vi "Begin.vi"(11 "Image Size":T1=enum."160x120") -> (0 "error out":errorcluster)   [LabVIEW 2011]
doc: "Called before other user functions, this VI is expected to open initial I/O refnums, load in file data, and do all program initialization. Notice that the <B>error out</B> terminal is simply used for data flow. Wiring it to other structures or subVIs ensures that this VI runs first."
uses:
  <vilib>/Rock Robotics/WPI/Camera/WPI_CameraImageSize.ctl
  <vilib>/Rock Robotics/WPI/Joystick/WPI_JoystickDeviceEnum.ctl
  <vilib>/Rock Robotics/WPI/Camera/WPI_CameraWhite Balance Values.ctl
  <vilib>/Rock Robotics/WPI/Camera/WPI_CameraExposure Values.ctl
  <vilib>/Rock Robotics/WPI/Camera/WPI_CameraFrameRate.ctl
  <vilib>/Rock Robotics/SystemInterfaces/DIO/FPGA_DIORelayChannel.ctl
  <vilib>/Rock Robotics/SystemInterfaces/DIO/FPGA_DIOChannel.ctl
  <vilib>/Rock Robotics/WPI/CAN/Jaguar/SubVIs/WPI_CANJaguar_ControlMode.ctl
  <vilib>/Rock Robotics/WPI/Solenoid/WPI_SolenoidChannel.ctl
  <vilib>/Rock Robotics/SystemInterfaces/Typedef/FPGA_TypedefAnalogModule.ctl
  <vilib>/Rock Robotics/SystemInterfaces/AI/FPGA_AIChannel.ctl
  <vilib>/Rock Robotics/SystemInterfaces/Typedef/FPGA_TypedefDigitalModule.ctl
  <vilib>/Rock Robotics/WPI/Encoder/WPI_EncoderType.ctl
  <vilib>/Rock Robotics/SystemInterfaces/DIO/FPGA_DIOPWMChannel.ctl
  <vilib>/Rock Robotics/SystemInterfaces/AI/FPGA_AIGyroChannel.ctl
  <vilib>/Rock Robotics/WPI/RobotDrive/WPI_RobotDriveOpen4MotorWithCANJaguar.vi
  <vilib>/Rock Robotics/WPI/MotorControl/WPI_MotorControlOpenCANJaguar.vi
  <vilib>/Rock Robotics/WPI/Counter/WPI_CounterDigitalInputToDigitalSource.vi
  <vilib>/Rock Robotics/WPI/Counter/WPI_CounterOpen Gear Tooth Sensor Mode.vi
  <vilib>/Rock Robotics/WPI/Solenoid/WPI_SolenoidOpenSingle.vi
  <vilib>/Rock Robotics/WPI/Compressor/WPI_CompressorGetSetRefNum.vi
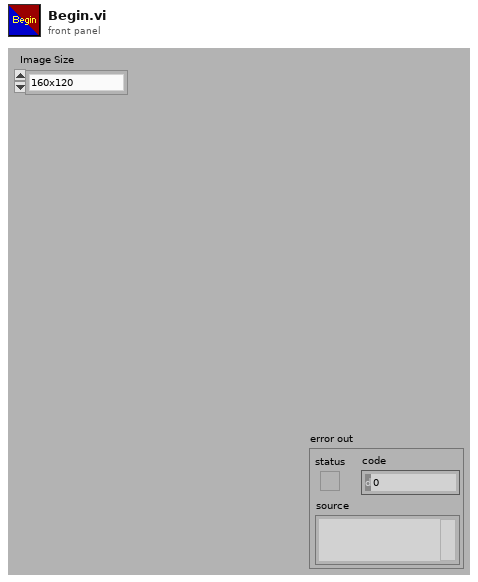
[diagram p1: front panel]
types:
  T1 = typedef "WPI_CameraImageSize.ctl" = enum16{"640x480", "320x240", "160x120"}
  T2 = typedef "WPI_SolenoidChannel.ctl" = enum8{"Solenoid 1", "Solenoid 2", "Solenoid 3", "Solenoid 4", "Solenoid 5", "Solenoid 6", "Solenoid 7", "Solenoid 8", "Invalid"}
  T3 = typedef "WPI_JoystickDeviceEnum.ctl" = enum16{"USB 1", "USB 2", "USB 3", "USB 4", "Kinect 1", "Kinect 2"}
  T4 = typedef "FPGA_AIGyroChannel.ctl" = enum8{"AI 1", "AI 2", "Invalid"}
  T5 = typedef "FPGA_DIOChannel.ctl" = enum8{"DIO 1", "DIO 2", "DIO 3", "DIO 4", "DIO 5", "DIO 6", "DIO 7", "DIO 8", "DIO 9", "DIO 10", "DIO 11", "DIO 12", "DIO 13", "DIO 14", "Invalid"}
  T6 = typedef "FPGA_DIOPWMChannel.ctl" = enum8{"PWM 1", "PWM 2", "PWM 3", "PWM 4", "PWM 5", "PWM 6", "PWM 7", "PWM 8", "PWM 9", "PWM 10", "Invalid"}
  T7 = typedef "WPI_EncoderType.ctl" = enum16{"1x", "2x", "4x"}
  T8 = typedef "FPGA_TypedefDigitalModule.ctl" = enum16{"Digital Module 1", "Digital Module 2"}
  T9 = typedef "FPGA_AIChannel.ctl" = enum8{"AI 1", "AI 2", "AI 3", "AI 4", "AI 5", "AI 6", "AI 7", "AI 8", "Invalid"}
  T10 = typedef "FPGA_TypedefAnalogModule.ctl" = enum16{"Analog Module 1", "Analog Module 2"}
  T11 = typedef "WPI_CANJaguar_ControlMode.ctl" = enum8{"Percent VBus", "Current", "Speed", "Position", "Voltage"}
  T12 = typedef "FPGA_DIORelayChannel.ctl" = enum8{"Relay 1", "Relay 2", "Relay 3", "Relay 4", "Relay 5", "Relay 6", "Relay 7", "Relay 8", "Invalid"}
  T13 = typedef "WPI_CameraFrameRate.ctl" = u32
  T14 = typedef "WPI_CameraExposure Values.ctl" = enum16{"Auto", "Flicker-free 50 Hz", "Flicker-free 60 Hz", "Hold current"}
  T15 = typedef "WPI_CameraWhite Balance Values.ctl" = enum16{"Auto", "Fixed indoor", "Fixed outdoor 1", "Fixed outdoor 2", "Fixed fluorescent 1", "Fixed fluorescent 2", "Hold current"}
  T16 = typedef "WPI_MotorControlDeviceRef.ctl" = cluster{"DeviceStatus":errorcluster, "Type":enum16{"PWM", "CAN"}, "PWM":cluster{"Digital Module":T8, "PWM Channel":T6, "DeadBand":T17}, "CAN":cluster{"Device Number":u8, "Control Mode":T11, "Semaphore":T18, "Max Vout":dbl}, "Invert":bool, "TransformRef":T19, "InvTransformRef":T19}
  T17 = typedef "WPI_PWMDeadband.ctl" = cluster{"Name":string, "maxPositivePwm":i32, "minPositivePwm":i32, "centerPwm":i32, "maxNegativePwm":i32, "minNegativePwm":i32, "angularRange":u16}
  T18 = typedef "Semaphore RefNum" = refnum<k1>
  T19 = typedef "WPI_PWMTransform_ConPane.ctl" = refnum<vi>
  T20 = typedef "WPI_DigitalInputDevRef.ctl" = cluster{"DevStatus":errorcluster, "DIO Channel":T5, "Digital Module":T8}
  T21 = typedef "WPI_JoystickDevRef.ctl" = cluster{"Device":T3}
  T22 = typedef "WPI_AnalogChannelDevRef.ctl" = cluster{"DevStatus":errorcluster, "Analog Module":T10, "Analog Channel":T9}
  T23 = typedef "WPI_RobotDriveDevRef.ctl" = cluster{"DevStatus":errorcluster, "Motors[]":T16[], "Square Inputs":bool, "Max Output":dbl, "Isochronous":bool}
  T24 = typedef "WPI_CameraDevRef.ctl" = cluster{"Camera Address":string, "CameraStatus":errorcluster, "Acquire Image Notifier":refnum<notifier>}
  T25 = typedef "WPI_SolenoidDevRef.ctl" = cluster{"DevStatus":errorcluster, "Solenoid Module":T26, "Forward Solenoid Channel":T2, "Reverse Solenoid Channel":T2}
  T26 = typedef "FPGA_TypedefSolenoidModule.ctl" = enum16{"Solenoid Module 1", "Solenoid Module 2"}
  T27 = typedef "FPGA_CounterEncoderSourceConvertionLVSourceType.ctl" = cluster{"DevStatus":errorcluster, "AnalogTriggerMode?":bool, "DigitalMode":cluster{"Digital Module":T8, "DIO Channel":T28}, "AnalogTriggerMode":cluster{"AnalogTriggerIndex":T29, "OutputType":T30}}
  T28 = typedef "FPGA_DIODigitalSourceChannel.ctl" = enum8{"DIO 1", "DIO 2", "DIO 3", "DIO 4", "DIO 5", "DIO 6", "DIO 7", "DIO 8", "DIO 9", "DIO 10", "DIO 11", "DIO 12", "DIO 13", "DIO 14", "Disabled"}
  T29 = typedef "FPGA_AnalogTriggerIndex.ctl" = enum8{"Trig 0", "Trig 1", "Trig 2", "Trig 3", "Trig 4", "Trig 5", "Trig 6", "Trig 7", "Invalid"}
  T30 = typedef "FPGA_AnalogTriggerOutType.ctl" = enum16{"InWindow", "TriggerState", "Rising", "Falling"}
  T31 = typedef "WPI_CompressorDevRef.ctl" = cluster{"DevStatus":errorcluster, "DigitalInputDevRef":T20, "RelayDevRef":T32}
  T32 = typedef "WPI_RelayDevRef.ctl" = cluster{"DevStatus":errorcluster, "Relay Channel":T12, "Digital Module":T8, "Relay Direction":T33}
  T33 = typedef "WPI_RelayDirection.ctl" = enum16{"Both directions", "Forward only", "Reverse only"}
  T34 = typedef "WPI_GyroDevRef.ctl" = cluster{"DevStatus":errorcluster, "Analog Module":T10, "Analog Channel":T9, "Offset":dbl, "Gain (VoltsPerDegree/Second)":dbl}
  T35 = typedef "WPI_CounterDevRef.ctl" = cluster{"DevStatus":errorcluster, "CntIndex":T36}
  T36 = typedef "FPGA_CounterCtrSystemIndex.ctl" = enum8{"Ctr 0", "Ctr 1", "Ctr 2", "Ctr 3", "Ctr 4", "Ctr 5", "Ctr 6", "Ctr 7", "Invalid"}
  T37 = typedef "WPI_ServoDeviceRef.ctl" = cluster{"DeviceStatus":errorcluster, "Digital Module":T8, "PWM Channel":T6, "DeadBand":T17}
  T38 = typedef "WPI_EncoderDevRef.ctl" = cluster{"DevStatus":errorcluster, "EncoderIndex":T39, "CounterIndex":T36, "DistancePerCount":dbl, "Decoding Type":T7}
  T39 = typedef "FPGA_EncoderIdx.ctl" = enum8{"Enc 0", "Enc 1", "Enc 2", "Enc 3", "Invalid"}
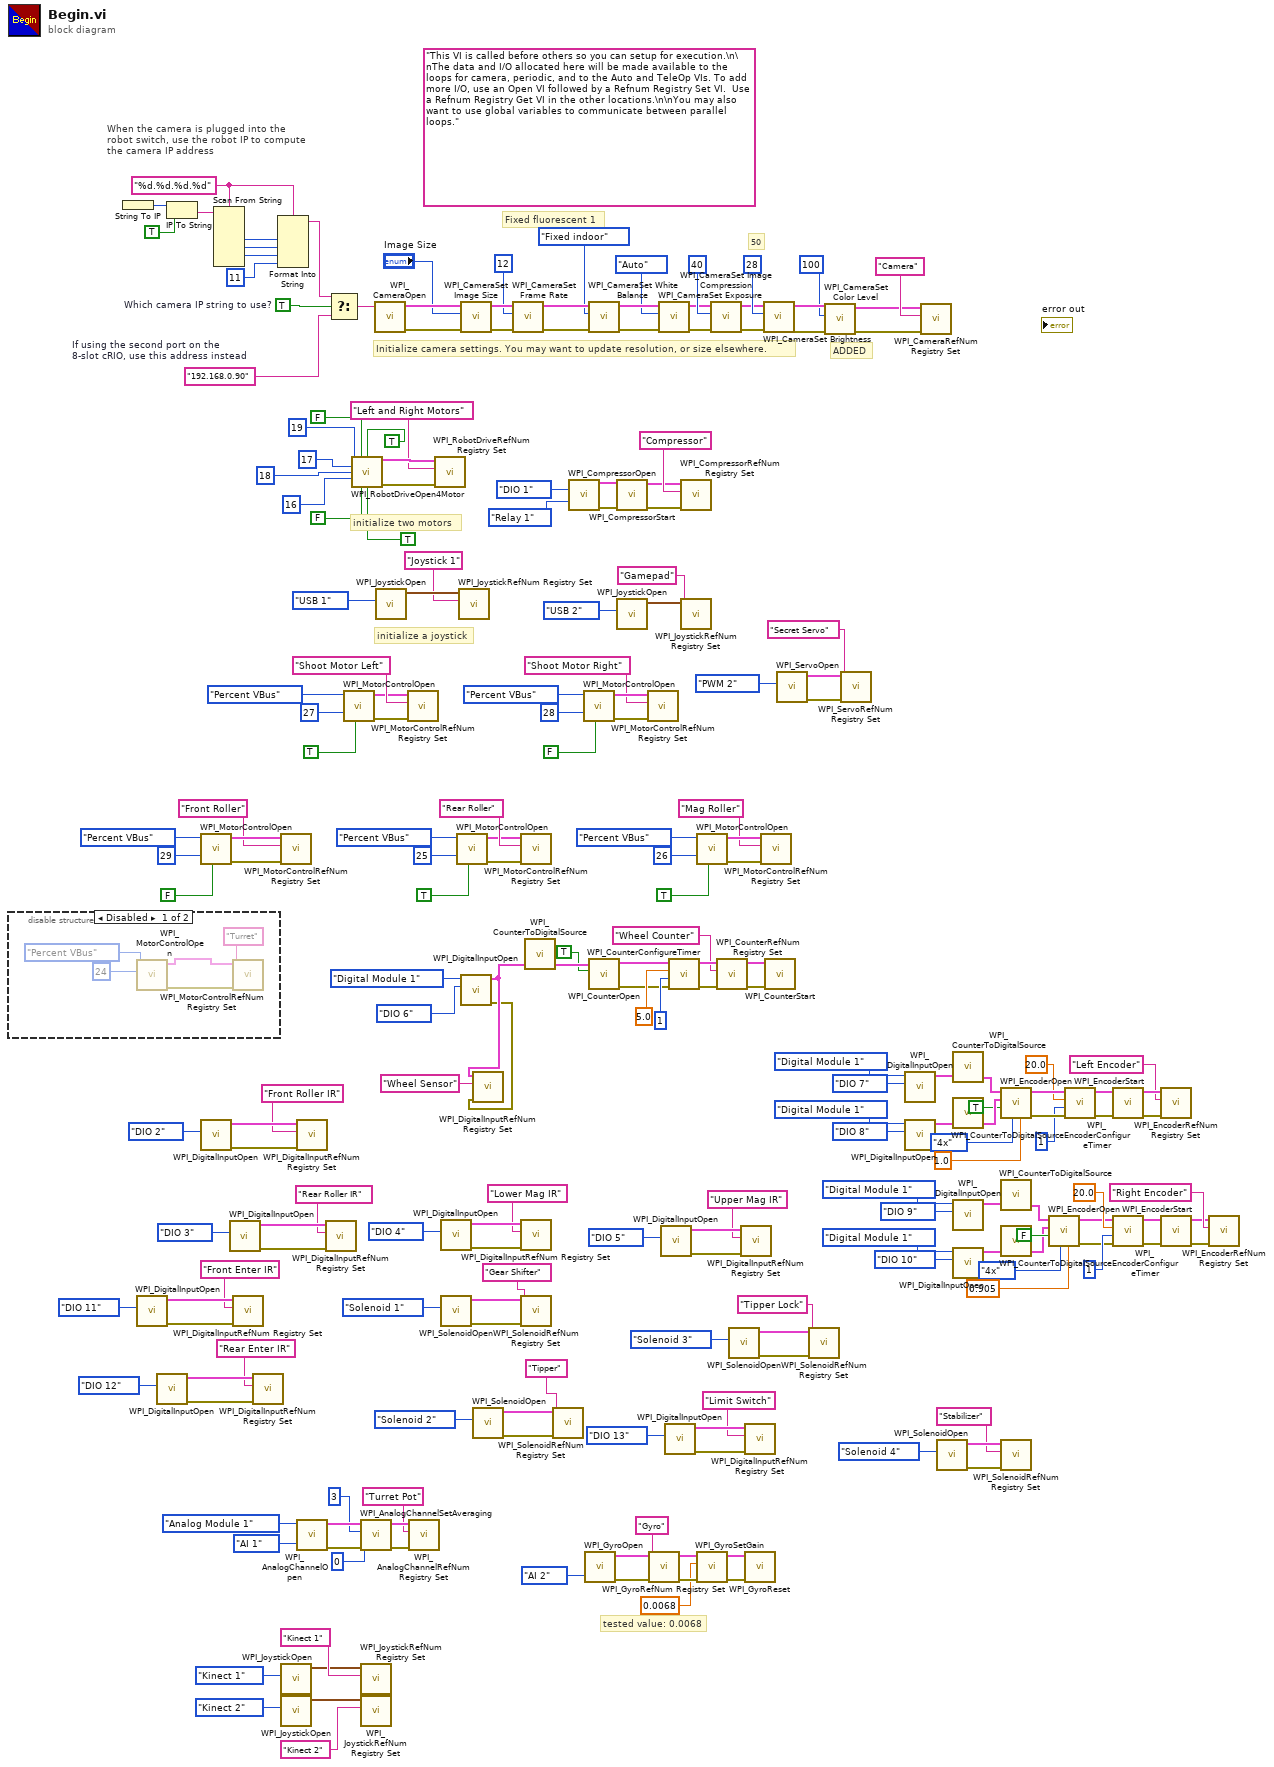
[diagram p0: block diagram]
diagram:
  w185 = TRUE  # Which camera IP string to use?
  w189 = "%d.%d.%d.%d" ("format string")
  (unwired) "This VI is called before others so you can setup for execution.\n\nThe data and I/O allocated here will be made available to the loops for camera, periodic, and to the Auto and TeleOp VIs. To add more I/O, use an Open VI followed by a Refnum Registry Set VI.  Use a Refnum Registry Get VI in the other locations.\n\nYou may also want to use global variables to communicate between parallel loops."
  w186 = "192.168.0.90"  # If using the second port on the 8-slot cRIO, use this address instead
  # "ADDED"
  # "50"
  # "Fixed fluorescent 1"
  # "tested value: 0.0068"
  # "initialize two motors"
  # "When the camera is plugged into the\nrobot switch, use the robot IP to compute\nthe camera IP address"
  # "initialize a joystick"
  # "Initialize camera settings. You may want to update resolution, or size elsewhere."
  n1 = disable-structure shown="Disabled" {
    frame Disabled {
      n2 = call-poly <vilib>:"WPI_MotorControlOpen.vi"("Device Number"=u8 24, "Control Mode"=WPI_CANJaguar_ControlMode."Percent VBus") -> ("error out"=w219:errorcluster, "MotorControlDeviceRef"=w221:T16)  [unwired: 8 in]
      n3 = call <vilib>:"WPI_MotorControlRefNum Registry Set.vi"("error in (no error)"=w219, "refnum name"="Turret", "MotorControlDevRef"=w221) -> ()  [unwired: 7 in, 2 out]
    }
    frame Enabled {
    }
  }
  n4 = String To IP() -> (0:w196:u32)  [unwired: 1 in]
  n5 = call <vilib>:"WPI_DigitalInputOpen.vi"("DIO Channel"=FPGA_DIOChannel."DIO 11") -> ("error out"=w33:errorcluster, "DigitalInputDevRef"=w36:T20)  [unwired: 9 in]
  n6 = call <vilib>:"WPI_DigitalInputOpen.vi"("DIO Channel"=FPGA_DIOChannel."DIO 12") -> ("error out"=w29:errorcluster, "DigitalInputDevRef"=w32:T20)  [unwired: 9 in]
  n7 = IP To String(1:TRUE ("dot notation? (F)"), 2:w196) -> (0:w194:string)
  n8 = call-poly <vilib>:"WPI_MotorControlOpen.vi"("Invert"=FALSE, "Device Number"=u8 29, "Control Mode"=WPI_CANJaguar_ControlMode."Percent VBus") -> ("error out"=w148:errorcluster, "MotorControlDeviceRef"=w149:T16)  [unwired: 7 in]
  n9 = call <vilib>:"WPI_DigitalInputOpen.vi"("DIO Channel"=FPGA_DIOChannel."DIO 2") -> ("error out"=w106:errorcluster, "DigitalInputDevRef"=w118:T20)  [unwired: 9 in]
  n10 = Scan From String(format string=w189, input string=w194) -> (output 1=w193:i32, output 2=w192:i32, output 3=w191:i32)  [unwired: 7 in, 3 out]
  n11 = call <vilib>:"WPI_DigitalInputOpen.vi"("DIO Channel"=FPGA_DIOChannel."DIO 3") -> ("error out"=w105:errorcluster, "DigitalInputDevRef"=w115:T20)  [unwired: 9 in]
  n12 = call <vilib>:"WPI_DigitalInputRefNum Registry Set.vi"("error in (no error)"=w33, "refnum name"="Front Enter IR", "DigitalInputDevRef"=w36) -> ()  [unwired: 7 in, 2 out]
  n13 = call <vilib>:"WPI_DigitalInputRefNum Registry Set.vi"("error in (no error)"=w29, "refnum name"="Rear Enter IR", "DigitalInputDevRef"=w32) -> ()  [unwired: 7 in, 2 out]
  n14 = Format Into String(format string=w189, w193, w192, w191, 11 ("Compression")) -> (resulting string=w187:string)  [unwired: 2 in, 1 out]
  n15 = call <vilib>:"WPI_MotorControlRefNum Registry Set.vi"("error in (no error)"=w148, "refnum name"="Front Roller", "MotorControlDevRef"=w149) -> ()  [unwired: 7 in, 2 out]
  n16 = call <vilib>:"WPI_JoystickOpen.vi"("JoystickDevice"=WPI_JoystickDeviceEnum."Kinect 1") -> ("JoystickDevRef"=w12:T21)  [unwired: 10 in]
  n17 = call <vilib>:"WPI_JoystickOpen.vi"("JoystickDevice"=WPI_JoystickDeviceEnum."Kinect 2") -> ("JoystickDevRef"=w15:T21)  [unwired: 10 in]
  n18 = call <vilib>:"WPI_DigitalInputRefNum Registry Set.vi"("error in (no error)"=w106, "refnum name"="Front Roller IR", "DigitalInputDevRef"=w118) -> ()  [unwired: 7 in, 2 out]
  n19 = call <vilib>:"WPI_AnalogChannelOpen.vi"("Analog Channel"=FPGA_AIChannel."AI 1", "Analog Module (Module 1)"=FPGA_TypedefAnalogModule."Analog Module 1") -> ("error out"=w86:errorcluster, "AIDeviceRef"=w87:T22)  [unwired: 8 in]
  n20 = call <vilib>:"WPI_DigitalInputRefNum Registry Set.vi"("error in (no error)"=w105, "refnum name"="Rear Roller IR", "DigitalInputDevRef"=w115) -> ()  [unwired: 7 in, 2 out]
  n21 = Select(t=w187, s=w185, f=w186) -> (s? t:f=w188:string)
  n22 = call-poly <vilib>:"WPI_MotorControlOpen.vi"("Invert"=TRUE, "Device Number"=u8 27, "Control Mode"=WPI_CANJaguar_ControlMode."Percent VBus") -> ("error out"=w164:errorcluster, "MotorControlDeviceRef"=w163:T16)  [unwired: 7 in]
  n23 = call-poly <vilib>:"WPI_RobotDriveOpen4Motor.vi"("Rear Left Motor"=u8 19, "Rear Left Motor Inverted"=FALSE, "Rear Right Motor Inverted"=TRUE ("Rear Left Motor Inverted"), "Rear Right Motor"=u8 17, "Front Left Motor"=u8 18, "Front Right Motor"=u8 16, "Front Left Motor Inverted"=FALSE, "Front Right Motor Inverted"=TRUE) -> ("RobotDriveDevRef"=w184:T23, "error out"=w182:errorcluster)  [unwired: 6 in]
  n24 = call <vilib>:"WPI_AnalogChannelSetAveraging.vi"("error in (no error)"=w86, "OversampleBits"=u8 0, "AverageBits"=u8 3, "AIDeviceRef"=w87) -> ("error out"=w83:errorcluster, "AIDeviceRef"=w82:T22)  [unwired: 6 in]
  n25 = call <vilib>:"WPI_JoystickRefNum Registry Set.vi"("refnum name"="Kinect 1", "JoystickDevRef"=w12) -> ()  [unwired: 8 in, 2 out]
  n26 = call <vilib>:"WPI_JoystickRefNum Registry Set.vi"("refnum name"="Kinect 2", "JoystickDevRef"=w15) -> ()  [unwired: 8 in, 2 out]
  n27 = call <vilib>:"WPI_CameraOpen.vi"("Camera Address"=w188) -> ("error out"=w207:errorcluster, "CameraDevRef"=w208:T24)  [unwired: 1 in, 8 out]
  n28 = call <vilib>:"WPI_JoystickOpen.vi"("JoystickDevice"=WPI_JoystickDeviceEnum."USB 1") -> ("JoystickDevRef"=w217:T21)  [unwired: 10 out]
  n29 = call <vilib>:"WPI_MotorControlRefNum Registry Set.vi"("error in (no error)"=w164, "refnum name"="Shoot Motor Left", "MotorControlDevRef"=w163) -> ()  [unwired: 7 in, 2 out]
  n30 = call <vilib>:"WPI_AnalogChannelRefNum Registry Set.vi"("error in (no error)"=w83, "refnum name"="Turret Pot", "AIDeviceRef"=w82) -> ()  [unwired: 7 in, 2 out]
  n31 = call <vilib>:"WPI_RobotDriveRefNum Registry Set.vi"("error in (no error)"=w182, "refnum name"="Left and Right Motors", "RobotDriveDevRef"=w184) -> ()  [unwired: 9 out]
  n32 = call <vilib>:"WPI_DigitalInputOpen.vi"("DIO Channel"=FPGA_DIOChannel."DIO 4") -> ("error out"=w104:errorcluster, "DigitalInputDevRef"=w112:T20)  [unwired: 9 in]
  n33 = call-poly <vilib>:"WPI_SolenoidOpen.vi"("Solenoid Channel"=WPI_SolenoidChannel."Solenoid 1") -> ("error out"=w100:errorcluster, "SolenoidDevRef"=w101:T25)  [unwired: 9 in]
  n34 = call-poly <vilib>:"WPI_MotorControlOpen.vi"("Invert"=TRUE, "Device Number"=u8 25, "Control Mode"=WPI_CANJaguar_ControlMode."Percent VBus") -> ("error out"=w143:errorcluster, "MotorControlDeviceRef"=w142:T16)  [unwired: 7 in]
  n35 = call <vilib>:"WPI_JoystickRefNum Registry Set.vi"("refnum name"="Joystick 1", "JoystickDevRef"=w217) -> ()  [unwired: 1 in, 9 out]
  n36 = call <vilib>:"WPI_CameraSet Image Size.vi"("error in (no error)"=w207, "Image Size"="Image Size", "CameraDevRef"=w208) -> ("error out"=w206:errorcluster, "CameraDevRef Out"=w209:T24)  [unwired: 7 out]
  n37 = call <vilib>:"WPI_DigitalInputOpen.vi"("DIO Channel"=FPGA_DIOChannel."DIO 6", "Digital Module (Module 1)"=FPGA_TypedefDigitalModule."Digital Module 1") -> ("error out"=w102:errorcluster, "DigitalInputDevRef"=w120:T20)  [unwired: 8 in]
  n38 = call <vilib>:"WPI_DigitalInputRefNum Registry Set.vi"("error in (no error)"=w102, "refnum name"="Wheel Sensor", "DigitalInputDevRef"=w120) -> ()  [unwired: 7 in, 2 out]
  n39 = call-poly <vilib>:"WPI_SolenoidOpen.vi"("Solenoid Channel"=WPI_SolenoidChannel."Solenoid 2") -> ("error out"=w98:errorcluster, "SolenoidDevRef"=w99:T25)  [unwired: 9 in]
  n40 = call <vilib>:"WPI_CameraSet Frame Rate.vi"("error in (no error)"=w206, "Frame Rate (fps)"=T13 12, "CameraDevRef"=w209) -> ("error out"=w205:errorcluster, "CameraDevRef Out"=w211:T24)  [unwired: 7 out]
  n41 = call <vilib>:"WPI_MotorControlRefNum Registry Set.vi"("error in (no error)"=w143, "refnum name"="Rear Roller", "MotorControlDevRef"=w142) -> ()  [unwired: 7 in, 2 out]
  n42 = call <vilib>:"WPI_DigitalInputRefNum Registry Set.vi"("error in (no error)"=w104, "refnum name"="Lower Mag IR", "DigitalInputDevRef"=w112) -> ()  [unwired: 7 in, 2 out]
  n43 = call <vilib>:"WPI_SolenoidRefNum Registry Set.vi"("error in (no error)"=w100, "refnum name"="Gear Shifter", "SolenoidDevRef"=w101) -> ()  [unwired: 7 in, 2 out]
  n44 = call-poly <vilib>:"WPI_CounterToDigitalSource.vi"("DigitalInputDevRef"=w120) -> ("Digital Source"=w131:T27)  [unwired: 6 in]
  n45 = call <vilib>:"WPI_SolenoidRefNum Registry Set.vi"("error in (no error)"=w98, "refnum name"="Tipper", "SolenoidDevRef"=w99) -> ()  [unwired: 7 in, 2 out]
  n46 = call <vilib>:"WPI_CompressorOpen.vi"("Pressure Switch DIO Channel"=FPGA_DIOChannel."DIO 1", "Relay Channel"=FPGA_DIORelayChannel."Relay 1") -> ("CompressorDevRef"=w169:T31, "error out"=w170:errorcluster)  [unwired: 12 in]
  n47 = call-poly <vilib>:"WPI_MotorControlOpen.vi"("Invert"=FALSE, "Device Number"=u8 28, "Control Mode"=WPI_CANJaguar_ControlMode."Percent VBus") -> ("error out"=w157:errorcluster, "MotorControlDeviceRef"=w158:T16)  [unwired: 7 in]
  n48 = call <vilib>:"WPI_GyroOpen.vi"("Analog Channel"=FPGA_AIGyroChannel."AI 2") -> ("error out"=w22:errorcluster, "GyroDevRef"=w24:T34)  [unwired: 8 in, 1 out]
  n49 = call <vilib>:"WPI_CameraSet White Balance.vi"("error in (no error)"=w205, "White Balance"=WPI_CameraWhite_Balance_Values."Fixed indoor", "CameraDevRef"=w211) -> ("error out"=w204:errorcluster, "CameraDevRef Out"=w210:T24)  [unwired: 7 out]
  n50 = call-poly <vilib>:"WPI_CounterOpen.vi"("Direction Sensitive"=TRUE ("High Pulse (T)"), "Source"=w131) -> ("error out"=w126:errorcluster, "CounterDevRef"=w127:T35)  [unwired: 8 in]
  n51 = call <vilib>:"WPI_CompressorStart.vi"("error in (no error)"=w170, "CompressorDevRef"=w169) -> ("error out"=w168:errorcluster, "CompressorDevRef"=w167:T31)  [unwired: 8 in]
  n52 = call <vilib>:"WPI_JoystickOpen.vi"("JoystickDevice"=WPI_JoystickDeviceEnum."USB 2") -> ("JoystickDevRef"=w153:T21)  [unwired: 10 in]
  n53 = call <vilib>:"WPI_MotorControlRefNum Registry Set.vi"("error in (no error)"=w157, "refnum name"="Shoot Motor Right", "MotorControlDevRef"=w158) -> ()  [unwired: 7 in, 2 out]
  n54 = call <vilib>:"WPI_GyroRefNum Registry Set.vi"("error in (no error)"=w22, "refnum name"="Gyro", "GyroDevRef"=w24) -> ("error out"=w20:errorcluster, "GyroDevRef"=w19:T34)  [unwired: 7 in]
  n55 = call <vilib>:"WPI_CameraSet Exposure.vi"("error in (no error)"=w204, "Exposure"=WPI_CameraExposure_Values."Auto", "CameraDevRef"=w210) -> ("error out"=w203:errorcluster, "CameraDevRef Out"=w213:T24)  [unwired: 7 out]
  n56 = call <vilib>:"WPI_DigitalInputOpen.vi"("DIO Channel"=FPGA_DIOChannel."DIO 5") -> ("error out"=w103:errorcluster, "DigitalInputDevRef"=w109:T20)  [unwired: 9 in]
  n57 = call <vilib>:"WPI_DigitalInputOpen.vi"("DIO Channel"=FPGA_DIOChannel."DIO 13") -> ("error out"=w27:errorcluster, "DigitalInputDevRef"=w28:T20)  [unwired: 9 in]
  n58 = call <vilib>:"WPI_CounterConfigureTimer.vi"("error in (no error)"=w126, "Number Samples to Average"=u8 1, "MaxPeriod (sec)"=5.0, "CounterDevRef in"=w127) -> ("error out"=w125:errorcluster, "CounterDevRef out"=w124:T35)  [unwired: 6 in]
  n59 = call <vilib>:"WPI_CompressorRefNum Registry Set.vi"("error in (no error)"=w168, "refnum name"="Compressor", "CompressorDevRef"=w167) -> ()  [unwired: 7 in, 2 out]
  n60 = call <vilib>:"WPI_JoystickRefNum Registry Set.vi"("refnum name"="Gamepad", "JoystickDevRef"=w153) -> ()  [unwired: 8 in, 2 out]
  n61 = call-poly <vilib>:"WPI_MotorControlOpen.vi"("Invert"=TRUE, "Device Number"=u8 26, "Control Mode"=WPI_CANJaguar_ControlMode."Percent VBus") -> ("error out"=w136:errorcluster, "MotorControlDeviceRef"=w137:T16)  [unwired: 7 in]
  n62 = call <vilib>:"WPI_GyroSetGain.vi"("error in (no error)"=w20, "Gain (VoltsPerDegree/Second)"=0.0068, "GyroDevRef"=w19) -> ("error out"=w6:errorcluster, "GyroDevRef"=w5:T34)  [unwired: 7 in]
  n63 = call <vilib>:"WPI_CameraSet Image Compression.vi"("error in (no error)"=w203, "Compression"=40, "CameraDevRef"=w213) -> ("error out"=w202:errorcluster, "CameraDevRef Out"=w212:T24)  [unwired: 7 out]
  n64 = call <vilib>:"WPI_CounterRefNum Registry Set.vi"("error in (no error)"=w125, "refnum name"="Wheel Counter", "CounterDevRef"=w124) -> ("error out"=w123:errorcluster, "CounterDevRef"=w122:T35)  [unwired: 7 in]
  n65 = call-poly <vilib>:"WPI_SolenoidOpen.vi"("Solenoid Channel"=WPI_SolenoidChannel."Solenoid 3") -> ("error out"=w96:errorcluster, "SolenoidDevRef"=w97:T25)  [unwired: 9 in]
  n66 = call <vilib>:"WPI_DigitalInputRefNum Registry Set.vi"("error in (no error)"=w103, "refnum name"="Upper Mag IR", "DigitalInputDevRef"=w109) -> ()  [unwired: 7 in, 2 out]
  n67 = call <vilib>:"WPI_DigitalInputRefNum Registry Set.vi"("error in (no error)"=w27, "refnum name"="Limit Switch", "DigitalInputDevRef"=w28) -> ()  [unwired: 7 in, 2 out]
  n68 = call <vilib>:"WPI_GyroReset.vi"("error in (no error)"=w6, "GyroDevRef"=w5) -> ()  [unwired: 8 in, 2 out]
  n69 = call <vilib>:"WPI_MotorControlRefNum Registry Set.vi"("error in (no error)"=w136, "refnum name"="Mag Roller", "MotorControlDevRef"=w137) -> ()  [unwired: 7 in, 2 out]
  n70 = call <vilib>:"WPI_CameraSet Brightness.vi"("error in (no error)"=w202, "Brightness"=28, "CameraDevRef"=w212) -> ("error out"=w11:errorcluster, "CameraDevRef Out"=w10:T24)  [unwired: 7 out]
  n71 = call <vilib>:"WPI_CounterStart.vi"("error in (no error)"=w123, "CounterDevRef in"=w122) -> ()  [unwired: 8 in, 2 out]
  n72 = call <vilib>:"WPI_ServoOpen.vi"("PWM Channel"=FPGA_DIOPWMChannel."PWM 2") -> ("error out"=w39:errorcluster, "ServoDeviceRef"=w40:T37)  [unwired: 9 in]
  n73 = call <vilib>:"WPI_SolenoidRefNum Registry Set.vi"("error in (no error)"=w96, "refnum name"="Tipper Lock", "SolenoidDevRef"=w97) -> ()  [unwired: 7 in, 2 out]
  n74 = call <vilib>:"WPI_CameraSet Color Level.vi"("error in (no error)"=w11, "Color Level"=100, "CameraDevRef"=w10) -> ("error out"=w8:errorcluster, "CameraDevRef Out"=w9:T24)  [unwired: 7 in]
  n75 = call <vilib>:"WPI_ServoRefNum Registry Set.vi"("error in (no error)"=w39, "refnum name"="Secret Servo", "ServoDeviceRef"=w40) -> ()  [unwired: 7 in, 2 out]
  n76 = call <vilib>:"WPI_DigitalInputOpen.vi"("DIO Channel"=FPGA_DIOChannel."DIO 7", "Digital Module (Module 1)"=FPGA_TypedefDigitalModule."Digital Module 1") -> ("DigitalInputDevRef"=w76:T20)  [unwired: 8 in, 1 out]
  n77 = call <vilib>:"WPI_DigitalInputOpen.vi"("DIO Channel"=FPGA_DIOChannel."DIO 8", "Digital Module (Module 1)"=FPGA_TypedefDigitalModule."Digital Module 1") -> ("DigitalInputDevRef"=w75:T20)  [unwired: 8 in, 1 out]
  n78 = call <vilib>:"WPI_CameraRefNum Registry Set.vi"("error in (no error)"=w8, "refnum name"="Camera", "CameraDevRef"=w9) -> ()  [unwired: 9 out]
  n79 = call-poly <vilib>:"WPI_SolenoidOpen.vi"("Solenoid Channel"=WPI_SolenoidChannel."Solenoid 4") -> ("error out"=w1:errorcluster, "SolenoidDevRef"=w3:T25)  [unwired: 9 in]
  n80 = call-poly <vilib>:"WPI_CounterToDigitalSource.vi"("DigitalInputDevRef"=w76) -> ("Digital Source"=w74:T27)  [unwired: 6 in]
  n81 = call-poly <vilib>:"WPI_CounterToDigitalSource.vi"("DigitalInputDevRef"=w75) -> ("Digital Source"=w73:T27)  [unwired: 6 in]
  n82 = call <vilib>:"WPI_DigitalInputOpen.vi"("DIO Channel"=FPGA_DIOChannel."DIO 9", "Digital Module (Module 1)"=FPGA_TypedefDigitalModule."Digital Module 1") -> ("DigitalInputDevRef"=w45:T20)  [unwired: 8 in, 1 out]
  n83 = call <vilib>:"WPI_DigitalInputOpen.vi"("DIO Channel"=FPGA_DIOChannel."DIO 10", "Digital Module (Module 1)"=FPGA_TypedefDigitalModule."Digital Module 1") -> ("DigitalInputDevRef"=w46:T20)  [unwired: 8 in, 1 out]
  n84 = call <vilib>:"WPI_EncoderOpen.vi"("DistancePerCount"=1.0, "Decoding Type"=WPI_EncoderType."4x", "Invert Direction (False)"=TRUE, "BSource"=w73, "ASource"=w74) -> ("error out"=w68:errorcluster, "EncoderDevRef"=w69:T38)  [unwired: 5 in]
  n85 = call-poly <vilib>:"WPI_CounterToDigitalSource.vi"("DigitalInputDevRef"=w45) -> ("Digital Source"=w47:T27)  [unwired: 6 in]
  n86 = call-poly <vilib>:"WPI_CounterToDigitalSource.vi"("DigitalInputDevRef"=w46) -> ("Digital Source"=w48:T27)  [unwired: 6 in]
  n87 = call <vilib>:"WPI_SolenoidRefNum Registry Set.vi"("error in (no error)"=w1, "refnum name"="Stabilizer", "SolenoidDevRef"=w3) -> ()  [unwired: 7 in, 2 out]
  n88 = call <vilib>:"WPI_EncoderOpen.vi"("DistancePerCount"=0.905, "Decoding Type"=WPI_EncoderType."4x", "Invert Direction (False)"=FALSE, "BSource"=w48, "ASource"=w47) -> ("error out"=w53:errorcluster, "EncoderDevRef"=w52:T38)  [unwired: 5 in]
  n89 = call <vilib>:"WPI_EncoderConfigureTimer.vi"("error in (no error)"=w68, "Number Samples to Average"=u8 1, "Minimum Rate"=20.0, "EncoderDevRef"=w69) -> ("error out"=w65:errorcluster, "EncoderDevRef"=w64:T38)  [unwired: 6 in]
  n90 = call <vilib>:"WPI_EncoderStart.vi"("error in (no error)"=w65, "EncoderDevRef"=w64) -> ("error out"=w63:errorcluster, "EncoderDevRef"=w62:T38)  [unwired: 8 in]
  n91 = call <vilib>:"WPI_EncoderConfigureTimer.vi"("error in (no error)"=w53, "Number Samples to Average"=u8 1, "Minimum Rate"=20.0, "EncoderDevRef"=w52) -> ("error out"=w56:errorcluster, "EncoderDevRef"=w57:T38)  [unwired: 6 in]
  n92 = call <vilib>:"WPI_EncoderRefNum Registry Set.vi"("error in (no error)"=w63, "refnum name"="Left Encoder", "EncoderDevRef"=w62) -> ()  [unwired: 7 in, 2 out]
  n93 = call <vilib>:"WPI_EncoderStart.vi"("error in (no error)"=w56, "EncoderDevRef"=w57) -> ("error out"=w58:errorcluster, "EncoderDevRef"=w59:T38)  [unwired: 8 in]
  n94 = call <vilib>:"WPI_EncoderRefNum Registry Set.vi"("error in (no error)"=w58, "refnum name"="Right Encoder", "EncoderDevRef"=w59) -> ()  [unwired: 7 in, 2 out]
